vi "Start Printing.vi"(8 "error in (no error)":errorcluster, 11 "Main.lvlib:Main.lvclass":refnum<class "Main.lvclass">) -> (0 "error out":errorcluster, 3 "Actor out":refnum<class "Actor.lvclass">)   [LabVIEW 2018, in "Main.lvlib" / "Main.lvclass"]
uses:
  Main.lvclass
  C:/Program Files/National Instruments/LabVIEW 2018/vi.lib/ActorFramework/Actor/Actor.lvclass
  <vilib>/ActorFramework/Actor/Actor.lvclass
  Main.lvclass/Main.ctl
  MFC Actor/MFC Messages/Change Setpoint Msg/Change Setpoint Msg.lvclass/Change Setpoint Msg.ctl
  <vilib>/ActorFramework/Message Enqueuer/Message Enqueuer.lvclass/Message Enqueuer.ctl
  Feeder Actor/Feeder Messages/Start Print Msg/Start Print Msg.lvclass/Start Print Msg.ctl
  <vilib>/ActorFramework/Message Enqueuer/Enqueue.vi
  MFC Actor/MFC Messages/Change Setpoint Msg/Change Setpoint Msg.lvclass
  C:/Program Files/National Instruments/LabVIEW 2018/vi.lib/ActorFramework/Message/Message.lvclass
  Feeder Actor/Feeder Messages/Start Print Msg/Start Print Msg.lvclass
  <vilib>/ActorFramework/Message Priority Queue/Priority Enqueue.vi
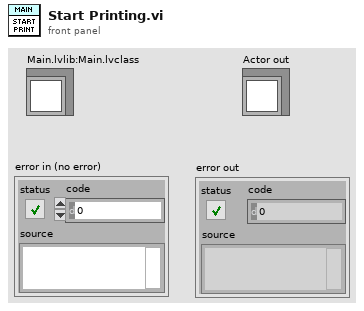
[diagram p1: front panel]
types:
  T1 = enum8{"Enabled", "Disabled", "Disabled and Grayed Out"}
  T2 = cluster{"Mixer Print Refnum":refnum<vi>, "Screw Print Refnum":refnum<vi>, "Inner Flow Print Refnum":refnum<vi>, "Outer Flow Print Refnum":refnum<vi>}
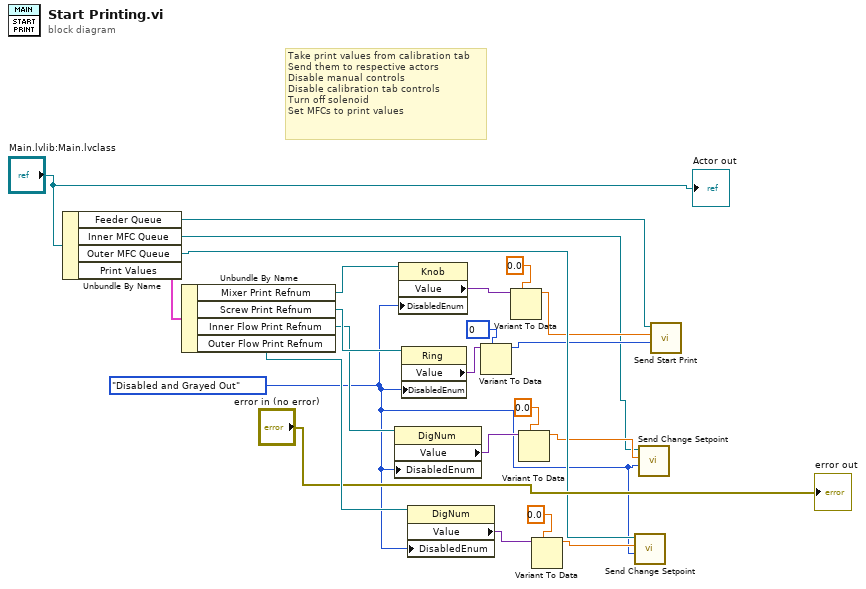
[diagram p0: block diagram]
diagram:
  w8 = u16 0 items=[""] ("Ring")
  w1 = T1."Disabled and Grayed Out" ("Disabled")
  # "Take print values from calibration tab\nSend them to respective actors\nDisable manual controls\nDisable calibration tab controls\nTurn off solenoid\nSet MFCs to print values"
  n1 = Unbundle By Name("Main.lvlib:Main.lvclass") -> ("Feeder Queue"=w7:refnum<class "Message Enqueuer.lvclass">, "Inner MFC Queue"=w3:refnum<class "Message Enqueuer.lvclass">, "Outer MFC Queue"=w12:refnum<class "Message Enqueuer.lvclass">, "Print Values"=w23:T2)
  n2 = Unbundle By Name(w23) -> ("Mixer Print Refnum"=w22:refnum<vi>, "Screw Print Refnum"=w21:refnum<vi>, "Inner Flow Print Refnum"=w20:refnum<vi>, "Outer Flow Print Refnum"=w19:refnum<vi>)
  n3 = property class="DigNum"(reference=w20, "DisabledEnum"=w1) -> ("Value"=w15:variant)  [unwired: 1 in, 2 out]
  n4 = property class="Knob"(reference=w22, "DisabledEnum"=w1) -> ("Value"=w10:variant)  [unwired: 1 in, 2 out]
  n5 = property class="Ring"(reference=w21, "DisabledEnum"=w1) -> ("Value"=w9:variant)  [unwired: 1 in, 2 out]
  n6 = property class="DigNum"(reference=w19, "DisabledEnum"=w1) -> ("Value"=w13:variant)  [unwired: 1 in, 2 out]
  n7 = Variant To Data(type=w8, Variant=w9) -> (data=w6:u16)  [unwired: 1 in, 1 out]
  n8 = Variant To Data(type=0.0, Variant=w10) -> (data=w5:dbl)  [unwired: 1 in, 1 out]
  n9 = Variant To Data(type=0.0, Variant=w15) -> (data=w4:dbl)  [unwired: 1 in, 1 out]
  n10 = Variant To Data(type=0.0, Variant=w13) -> (data=w2:dbl)  [unwired: 1 in, 1 out]
  n11 = call "Send Change Setpoint.vi"("Disabled"=w1, "Setpoint"=w2, "Message Enqueuer in"=w12) -> ()  [unwired: 7 in, 2 out]
  n12 = call "Send Change Setpoint.vi"("Disabled"=w1, "Setpoint"=w4, "Message Enqueuer in"=w3) -> ()  [unwired: 7 in, 2 out]
  n13 = call "Send Start Print.vi"("Screw"=w6, "Mixer"=w5, "Message Enqueuer"=w7) -> ()  [unwired: 7 in, 2 out]
  "Actor out" <- "Main.lvlib:Main.lvclass"
  "error out" <- "error in (no error)"
